vi "3_3_Elipse.vi"() -> ()   [LabVIEW 2020]
panel:
  out "Graficador de Elipse":cluster{dbl[], dbl[]}(graph)
  in  "R":dbl
  in  "B":dbl
  in  "A":dbl
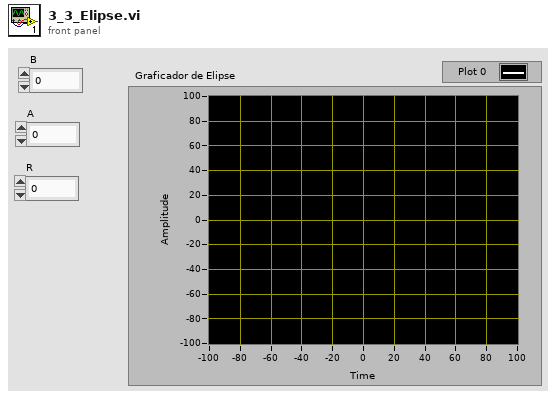
[diagram p1: front panel]
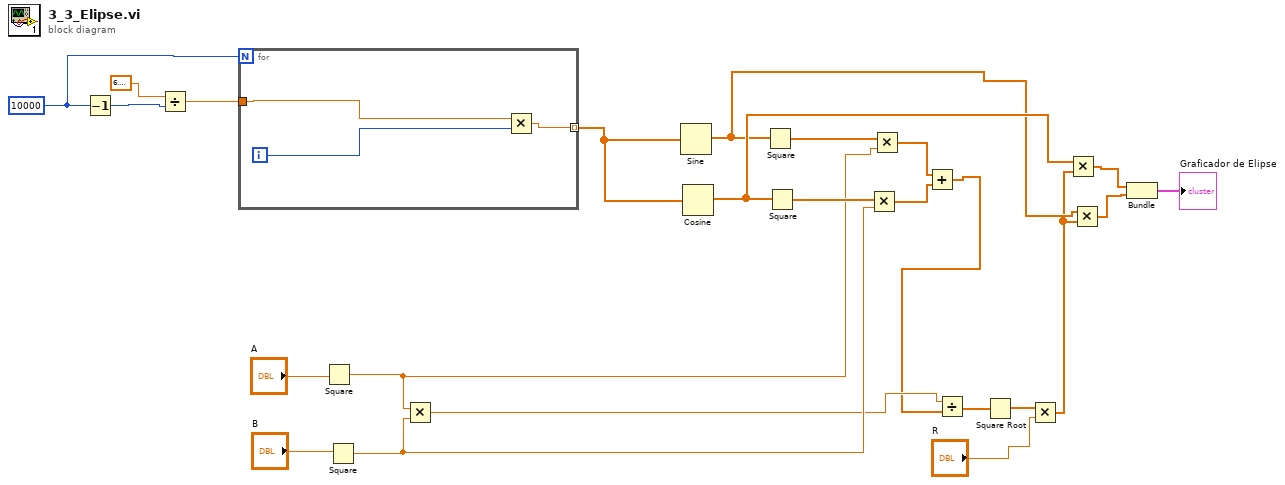
[diagram p0: block diagram]
diagram:
  w22 = 10000
  n1 = Decrement(x=w22) -> (x-1=w24:i32)
  n2 = Divide(x=6.283185307179586, y=w24) -> (x/y=w21:dbl)
  n3 = for {
    N: w22 -> [_]
    tunnel: w21 -> [w27]
    tunnel: [w25] -> w18 mode=indexing
    i -> [w26]
    n4 = Multiply(x=w27, y=w26) -> (x*y=w25:dbl)
  }
  n5 = Square(x="A") -> (x^2=w15:dbl)
  n6 = Square(x="B") -> (x^2=w14:dbl)
  n7 = Multiply(x=w15, y=w14) -> (x*y=w11:dbl)
  n8 = Sine(x=w18) -> (sin(x)=w8:dbl[])
  n9 = Cosine(x=w18) -> (cos(x)=w9:dbl[])
  n10 = Square(x=w8) -> (x^2=w17:dbl[])
  n11 = Square(x=w9) -> (x^2=w16:dbl[])
  n12 = Multiply(x=w16, y=w14) -> (x*y=w13:dbl[])
  n13 = Multiply(x=w17, y=w15) -> (x*y=w12:dbl[])
  n14 = Add(x=w12, y=w13) -> (x+y=w10:dbl[])
  n15 = Divide(x=w11, y=w10) -> (x/y=w2:dbl[])
  n16 = Square Root(x=w2) -> (sqrt(x)=w3:dbl[])
  n17 = Multiply(x=w3, y="R") -> (x*y=w1:dbl[])
  n18 = Multiply(x=w9, y=w1) -> (x*y=w7:dbl[])
  n19 = Multiply(x=w8, y=w1) -> (x*y=w6:dbl[])
  n20 = Bundle(w7, w6) -> (→"Graficador de Elipse":cluster{dbl[], dbl[]})  [unwired: 1 in]
